vi "Close.vi"(8 "error in (no error)":errorcluster, 11 "NetworkStreamReader in":refnum<class "NetworkStreamReader.lvclass">) -> (0 "error out":errorcluster, 3 "NetworkStreamReader out":refnum<class "NetworkStreamReader.lvclass">)   [LabVIEW 2011, in "NetworkStreamReader.lvclass"]
doc: "This VI closes references internal to the NetworkStreamReader object. This allows memory to be cleaned up effectively."
uses:
  NetworkStreamReader.lvclass
  NetworkStreamReader.lvclass/NetworkStreamReader.ctl
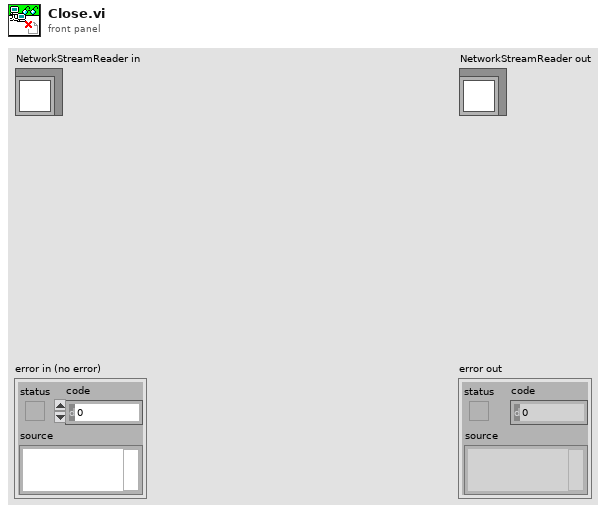
[diagram p1: front panel]
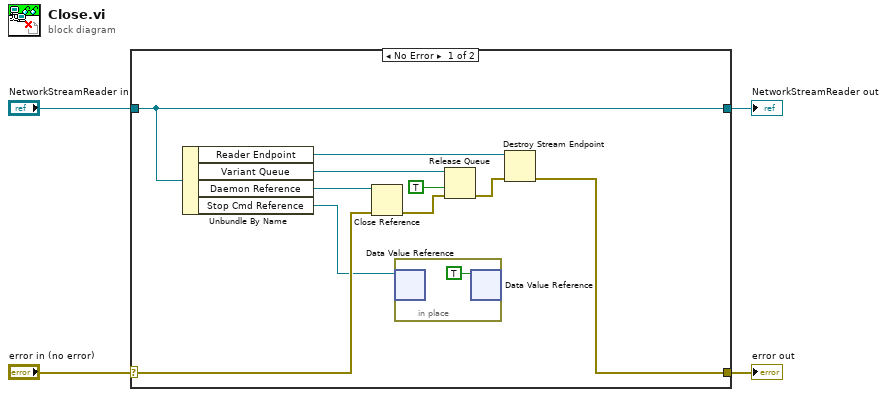
[diagram p0: block diagram]
diagram:
  n1 = case shown="No Error" "error in (no error)" {
    selector: "error in (no error)" -> [w12 w17]
    tunnel: [w7 w17] -> w3
    tunnel: [w14 w16] -> w1
    tunnel: "NetworkStreamReader in" -> [w14 w16]
    frame No Error {
      n2 = Unbundle By Name(w14) -> ("Reader Endpoint"=w9:refnum<k21>, "Variant Queue"=w11:refnum<queue>, "Daemon Reference"=w13:refnum<vi>, "Stop Cmd Reference"=w5:refnum<data-value>)
      n3 = Close Reference(reference=w13, error in (no error)=w12) -> (error out=w10:errorcluster)
      n4 = in-place {
        n5 = in-place-dvr #1(w5) -> ()  [unwired: 2 out]
        n6 = in-place-dvr #1(TRUE ("data value")) -> ()  [unwired: 2 out]
      }
      n7 = Release Queue(queue=w11, force destroy? (F)=TRUE, error in (no error)=w10) -> (error out=w8:errorcluster)  [unwired: 2 out]
      n8 = Destroy Stream Endpoint(8:w8, 11:w9) -> (0:w7:errorcluster)
    }
    frame Error {
    }
  }
  "error out" <- w3
  "NetworkStreamReader out" <- w1
